vi "test_OpticalLevel_fpga.vi"() -> ()   [LabVIEW 2020]
uses:
  <vilib>/rvi/Emulation/niFpgaGetClockAttributes.vi
  <vilib>/rvi/Emulation/niFpgaSctlEmulationGetInTimedLoop.vi
  <vilib>/rvi/Emulation/niFpgaEmulationReportErrorSimple.vi
  <vilib>/rvi/eio/common/nirviEmuTemplateMethod_errors.vi
  <vilib>/rvi/interface/RandomDataEmulation/nirviRandomDataMultiElementFPGAFIFO.vi
  <instcachedir>/0/nirviRandomDataMultiElementFPGAFIFO_3E9965BA1FAD4E7B8DABA31768A09B1F.lvgen/nirviRandomDataMultiElementFPGAFIFO_3E9965BA1FAD4E7B8DABA31768A09B1F_001.vi
  <vilib>/rvi/interface/RandomDataEmulation/niFpgaRandomDataHandleErrors.vi
  <vilib>/rvi/Emulation/niFpgaCriticalErrorInLSC.vi
  <vilib>/eio/EIONode/EIONode.xnode
  <vilib>/rvi/DataTransferAndStorage/Container/XNode/niFpgaContainer.xnode
  <vilib>/rvi/interface/RandomDataEmulation/nirviRandomDataFpgaMultiElementTemplate.vi
panel:
  in  "decimation":i16
  in  "stop":bool
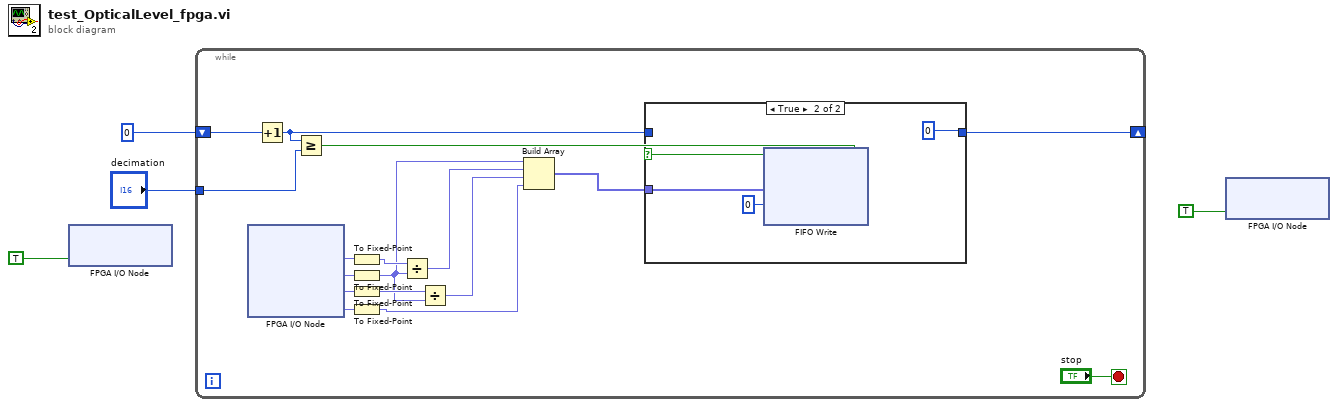
[diagram p0: block diagram]
diagram:
  n1 = xnode "FPGA I/O Node"("Mod1/Start"=TRUE ("Mod2/Start")) -> ()  [unwired: 2 in, 2 out]
  n2 = while {
    shift-right: [w16] -> _
    shift-left: i16 0 -> [w20]
    tunnel: "decimation" -> [w19]
    stop <- "stop" stop-if-true
    n3 = xnode "FPGA I/O Node"() -> ("Mod1/AI0"=w14:fxp<+/-,24,5>, "Mod1/AI1"=w13:fxp<+/-,24,5>, "Mod1/AI2"=w11:fxp<+/-,24,5>, "Mod1/AI3"=w6:fxp<+/-,24,5>)  [unwired: 5 in, 5 out]
    n4 = Increment(x=w20) -> (x+1=w17:i16)
    n5 = Greater Or Equal?(x=w17, y=w19) -> (x >= y?=w18:bool)
    n6 = To Fixed-Point(number=w14) -> (fixed-point=w12:fxp<+/-,64,20>)  [unwired: 1 in]
    n7 = To Fixed-Point(number=w13) -> (fixed-point=w9:fxp<+/-,64,20>)  [unwired: 1 in]
    n8 = To Fixed-Point(number=w11) -> (fixed-point=w10:fxp<+/-,64,20>)  [unwired: 1 in]
    n9 = To Fixed-Point(number=w6) -> (fixed-point=w5:fxp<+/-,64,20>)  [unwired: 1 in]
    n10 = Divide(x=w12, y=w9) -> (x/y=w8:fxp<+/-,64,20>)
    n11 = Divide(x=w10, y=w9) -> (x/y=w7:fxp<+/-,64,20>)
    n12 = Build Array(w9, w8, w7, w5) -> (w15:fxp<+/-,64,20>[])
    n13 = case shown="True" w18 {
      tunnel: w17 -> [w22 _]
      tunnel: [w22 i16 0] -> w16
      tunnel: w15 -> [_ w23]
      frame False {
      }
      frame True {
        n14 = xnode ("FIFO Write")("Element"=w23, "Timeout"=0) -> ()  [unwired: 2 in, 3 out]
      }
    }
  }
  n15 = xnode "FPGA I/O Node"("Mod1/Stop"=TRUE ("Mod2/Stop")) -> ()  [unwired: 2 in, 2 out]
